vi "dispose_.vi"(8 "error in (no error)":errorcluster, 11 "Lua Thread in":refnum<class "Lua Thread.lvclass">) -> (0 "error out":errorcluster)   [LabVIEW 2020, in "Lua for LabVIEW.lvlib" / "Lua Thread.lvclass"]
uses:
  Lua Thread.lvclass
  C:/Users/Nicholas Folse/Documents/workspace/github-tauterra.llc/Lua for LabVIEW/Lua for LabVIEW/Lua/Lua.lvclass
  Lua Thread.lvclass/Lua Thread.ctl
  Lua/Lua.lvclass
  C:/Users/Nicholas Folse/Documents/workspace/github-tauterra.llc/Lua for LabVIEW/Lua for LabVIEW/Disposable/Disposable.lvclass
  C:/Users/Nicholas Folse/Documents/workspace/github-tauterra.llc/Lua for LabVIEW/Lua for LabVIEW/Lua Thread/Lua Thread.lvclass
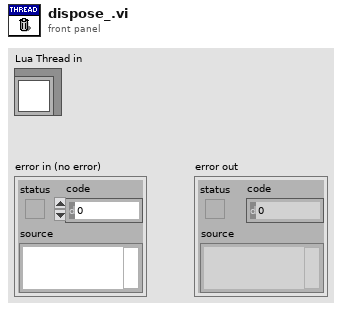
[diagram p1: front panel]
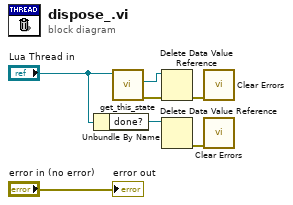
[diagram p0: block diagram]
diagram:
  n1 = Unbundle By Name("Lua Thread in") -> ("done?"=w2:refnum<data-value>)
  n2 = call "get_this_state.vi"("Lua in"="Lua Thread in") -> ("error out"=w6:errorcluster, "this state"=w7:refnum<data-value>)  [unwired: 8 in, 1 out]
  n3 = Delete Data Value Reference(data value reference=w7, error in=w6) -> (error out=w5:errorcluster)  [unwired: 1 out]
  n4 = Delete Data Value Reference(data value reference=w2) -> (error out=w1:errorcluster)  [unwired: 1 in, 1 out]
  n5 = call <vilib>:"Clear Errors.vi"("error in (no error)"=w5) -> ()  [unwired: 5 in, 2 out]
  n6 = call <vilib>:"Clear Errors.vi"("error in (no error)"=w1) -> ()  [unwired: 5 in, 2 out]
  "error out" <- "error in (no error)"
